vi "Turret_Correct_Sensor_Position.vi"(1 "error in (no error)":errorcluster, 4 "PhoenixMotorControlDevRef":T1) -> ()   [LabVIEW 2019]
uses:
  <vilib>/Rock Robotics/WPI/MotorControl/WPI_MotorControlDeviceRef.ctl
  <vilib>/Rock Robotics/WPI/MotorControl/WPI_MotorControlType.ctl
  <vilib>/Rock Robotics/SystemInterfaces/DIO/FPGA_DIOPWMChannel.ctl
  <vilib>/Rock Robotics/WPI/PWM/WPI_PWMDeadband.ctl
  <vilib>/Rock Robotics/SystemInterfaces/DIO/FPGA_DIOChannel.ctl
  Globals/Sensor_Values.vi
  Globals/Turret_Globals.vi
panel:
  out "final position":dbl
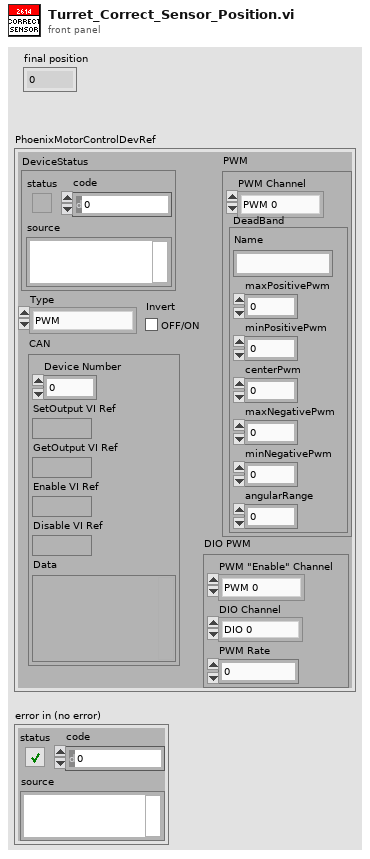
[diagram p1: front panel]
types:
  T1 = typedef "WPI_MotorControlDeviceRef.ctl" = cluster{"DeviceStatus":errorcluster, "Type":T2, "PWM":cluster{"PWM Channel":T3, "DeadBand":T4}, "CAN":cluster{"Device Number":u8, "SetOutput VI Ref":variant, "GetOutput VI Ref":variant, "Enable VI Ref":variant, "Disable VI Ref":variant, "Data":variant}, "Invert":bool, "DIO PWM":cluster{"PWM \"Enable\" Channel":T3, "DIOChannel":T5, "PWM Rate":dbl}}
  T2 = typedef "WPI_MotorControlType.ctl" = enum16{"PWM", "CAN", "DIO PWM"}
  T3 = typedef "FPGA_DIOPWMChannel.ctl" = enum8{"PWM 0", "PWM 1", "PWM 2", "PWM 3", "PWM 4", "PWM 5", "PWM 6", "PWM 7", "PWM 8", "PWM 9", "PWM MXP 0", "PWM MXP 1", "PWM MXP 2", "PWM MXP 3", "PWM MXP 4", "PWM MXP 5", "PWM MXP 6", "PWM MXP 7", "PWM MXP 8", "PWM MXP 9", "Invalid"}
  T4 = typedef "WPI_PWMDeadband.ctl" = cluster{"Name":string, "maxPositivePwm":i32, "minPositivePwm":i32, "centerPwm":i32, "maxNegativePwm":i32, "minNegativePwm":i32, "angularRange":u16}
  T5 = typedef "FPGA_DIOChannel.ctl" = enum8{"DIO 0", "DIO 1", "DIO 2", "DIO 3", "DIO 4", "DIO 5", "DIO 6", "DIO 7", "DIO 8", "DIO 9", "DIO MXP 0", "DIO MXP 1", "DIO MXP 2", "DIO MXP 3", "DIO MXP 4", "DIO MXP 5", "DIO MXP 6", "DIO MXP 7", "DIO MXP 8", "DIO MXP 9", "DIO MXP 10", "DIO MXP 11", "DIO MXP 12", "DIO MXP 13", "DIO MXP 14", "DIO MXP 15", "SPI Port CS1", "SPI Port CS2", "SPI Port CS3", "SPI Port MISO", "SPI Port MOSI", "Invalid"}
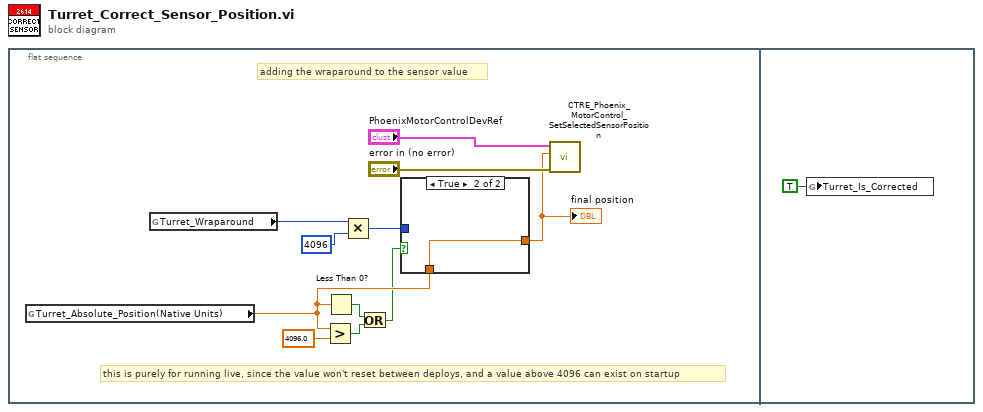
[diagram p0: block diagram]
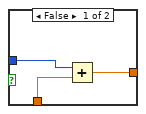
[diagram p2: hidden frame]
diagram:
  n1 = flat-sequence {
    frame #0 {
      # "this is purely for running live, since the value won't reset between deploys, and a value above 4096 can exist on startup"
      # "adding the wraparound to the sensor value"
      n2 = global read "Sensor_Values.vi" "Turret_Absolute_Position(Native Units)"() -> (w4:dbl)
      n3 = global read "Turret_Globals.vi" "Turret_Wraparound"() -> (w5:i32)
      n4 = Greater?(x=w4, y=4096.0) -> (0:w1:bool)
      n5 = Less Than 0?(x=w4) -> (x < 0?=w2:bool)
      n6 = Multiply(x=w5, y=4096) -> (x*y=w9:i32)
      n7 = Or(x=w2, y=w1) -> (x .or. y?=w3:bool)
      n8 = case shown="True" w3 {
        tunnel: w9 -> [w14 _]
        tunnel: [w13 w15] -> w8
        tunnel: w4 -> [w12 w15]
        frame False {
          n9 = Add(x=w14, y=w12) -> (x+y=w13:dbl)
        }
        frame True {
        }
      }
      "final position" <- w8
      n10 = call <vilib>:"CTRE_Phoenix_MotorControl_SetSelectedSensorPosition.vi"("error in (no error)"="error in (no error)", "New Sensor Position"=w8, "PhoenixMotorControlDevRef"="PhoenixMotorControlDevRef") -> ()  [unwired: 7 in, 2 out]
    }
    frame #1 {
      n11 = global write "Turret_Globals.vi" "Turret_Is_Corrected"(TRUE ("Turret_Is_Corrected")) -> ()
    }
  }
